vi "Day 6-1.vi"() -> ()   [LabVIEW 2019, in "Day 6.lvlib"]
uses:
  Day 6.lvlib
panel:
  out "Final number fo fishes":i32
  out "Final State":u32[](array[numeric])
  in  "String":string="3,5,1,2,5,4,1,5,1,2,5,5,1,3,1,5,1,3,2,1,5,1,1,1,2,3,1,3,1,2,1,1,5,1,5,4,5,5,3,3,1,5,1,1,5,5,1,3,5,5,3,2,2,4,1,5,3,4,2,5,4,1,2,2,5,1,1,2,4,4,1,3,1,3,1,1,2,2,1,1,5,1,1,4,4,5,5,1,2,1,4,1,1,4,4,3,4,2,2,3,3,2,1,3,3,2,1,1,1,2,1,4,2,2,1,5,5,3,4,5,5,2,5,2,2,5,3,3,1,2,4,2,1,5,1,1,2,3,5,5,1,1,5,5,1,4,5,3,5,2,3,2,4,3,1,4,2,5,1,3,2,1,1,3,4,2,1,1,1,1,2,1,4,3,1,3,1,2,4,1,2,4,3,2,3,5,5,3,3,1,2,3,4,5,2,4,5,1,1,1,4,5,3,5,3,5,1,1,5,1,5,3,1,2,3,4,1,1,4,1,2,4,1,5,4,1,5,4,2,1,5,2,1,3,5,5,4,5,5,1,1,4,1,2,3,5,3,3,1,1,1,4,3,1,1,4,1,5,3,5,1,4,2,5,1,1,4,4,4,2,5,1,2,5,2,1,3,1,5,1,2,1,1,5,2,4,2,1,3,5,5,4,1,1,1,5,5,2,1,1"
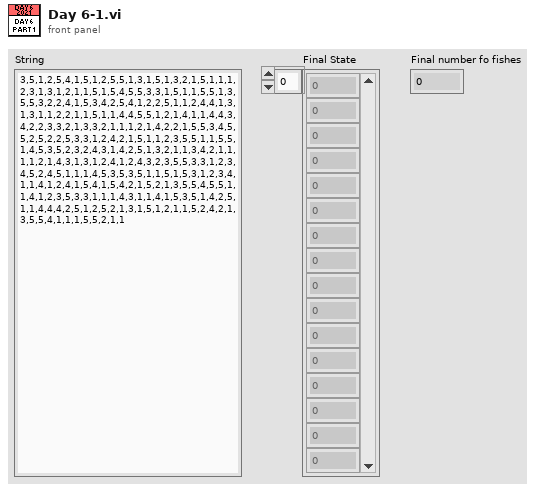
[diagram p1: front panel]
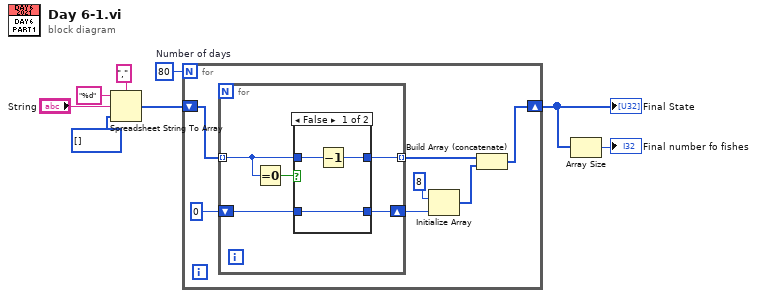
[diagram p0: block diagram]
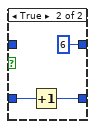
[diagram p2: hidden frame]
diagram:
  w4 = 80  # Number of days
  n1 = Spreadsheet String To Array(delimiter (Tab)=",", format string="%d", spreadsheet string="String", array type (2D Dbl)=u32[] []) -> (array=w3:u32[])
  n2 = for {
    N: w4 -> [_]
    shift-right: [w9] -> w2
    shift-left: w3 -> [w15]
    n3 = for {
      tunnel: w15 -> [w19] mode=indexing
      tunnel: [w20] -> w11 mode=indexing
      shift-right: [w16] -> w12
      shift-left: u32 0 -> [w17]
      n4 = Equal To 0?(x=w19) -> (x = 0?=w18:bool)
      n5 = case shown="False" w18 {
        tunnel: [w23 u32 6] -> w20
        tunnel: w19 -> [w22 _]
        tunnel: w17 -> [w21 w25]
        tunnel: [w21 w24] -> w16
        frame False {
          n6 = Decrement(x=w22) -> (x-1=w23:u32)
        }
        frame True {
          n7 = Increment(x=w25) -> (x+1=w24:u32)
        }
      }
    }
    n8 = Initialize Array(u32 8, w12) -> (w10:u32[])
    n9 = Build Array (concatenate)(w11, w10) -> (w9:u32[])
  }
  "Final State" <- w2
  n10 = Array Size(array=w2) -> (size(s)=→"Final number fo fishes":i32)
